vi "电机定位1.1（备份）.vi"(0 "VISA I":refnum<visa-resource-name>, 1 "等待时间(ms)":u32=40, 2 "细分设置":dbl=8.0, 3 "电机急停":bool, 4 "X":dbl, 5 "精度":dbl=0.001, 6 "pulDDR2Length":u32, 8 "hDevice":i32, 10 "M-length":dbl, 12 "N-length":dbl) -> (13 "hDevice out":i32, 14 "VISA O":refnum<visa-resource-name>, 18 "X":dbl, 19 "Y":dbl)   [LabVIEW 2016]
panel:
  out "幅频谱":dbl[](graph)
  out "时域谱":dbl[](graph)
  in  "查询信号":bool
  in  "Y":dbl
  in  "确定":bool
  in  "ESC":bool
  # "时域谱"
  # "频域谱"
  # "目标位置"
  # "实时位置"
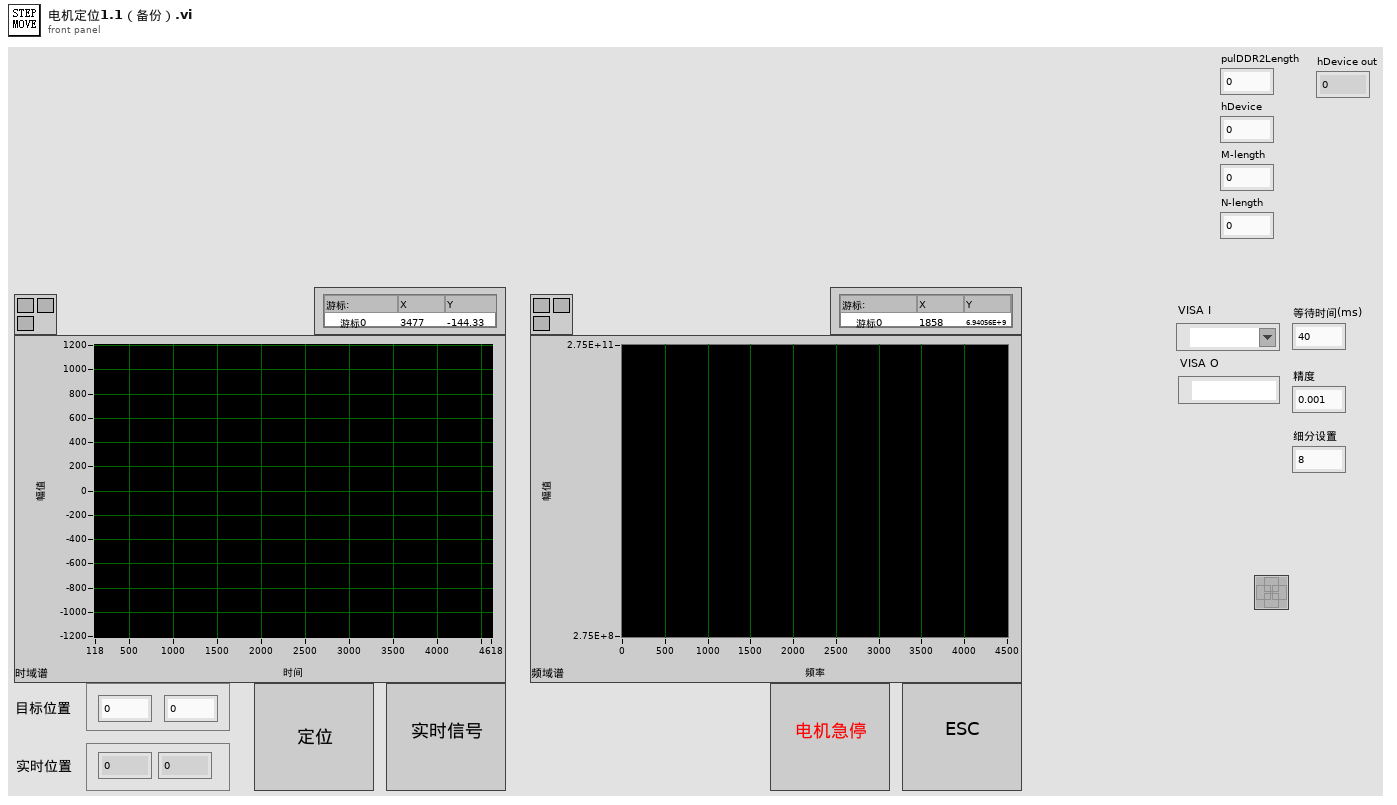
[diagram p1: front panel]
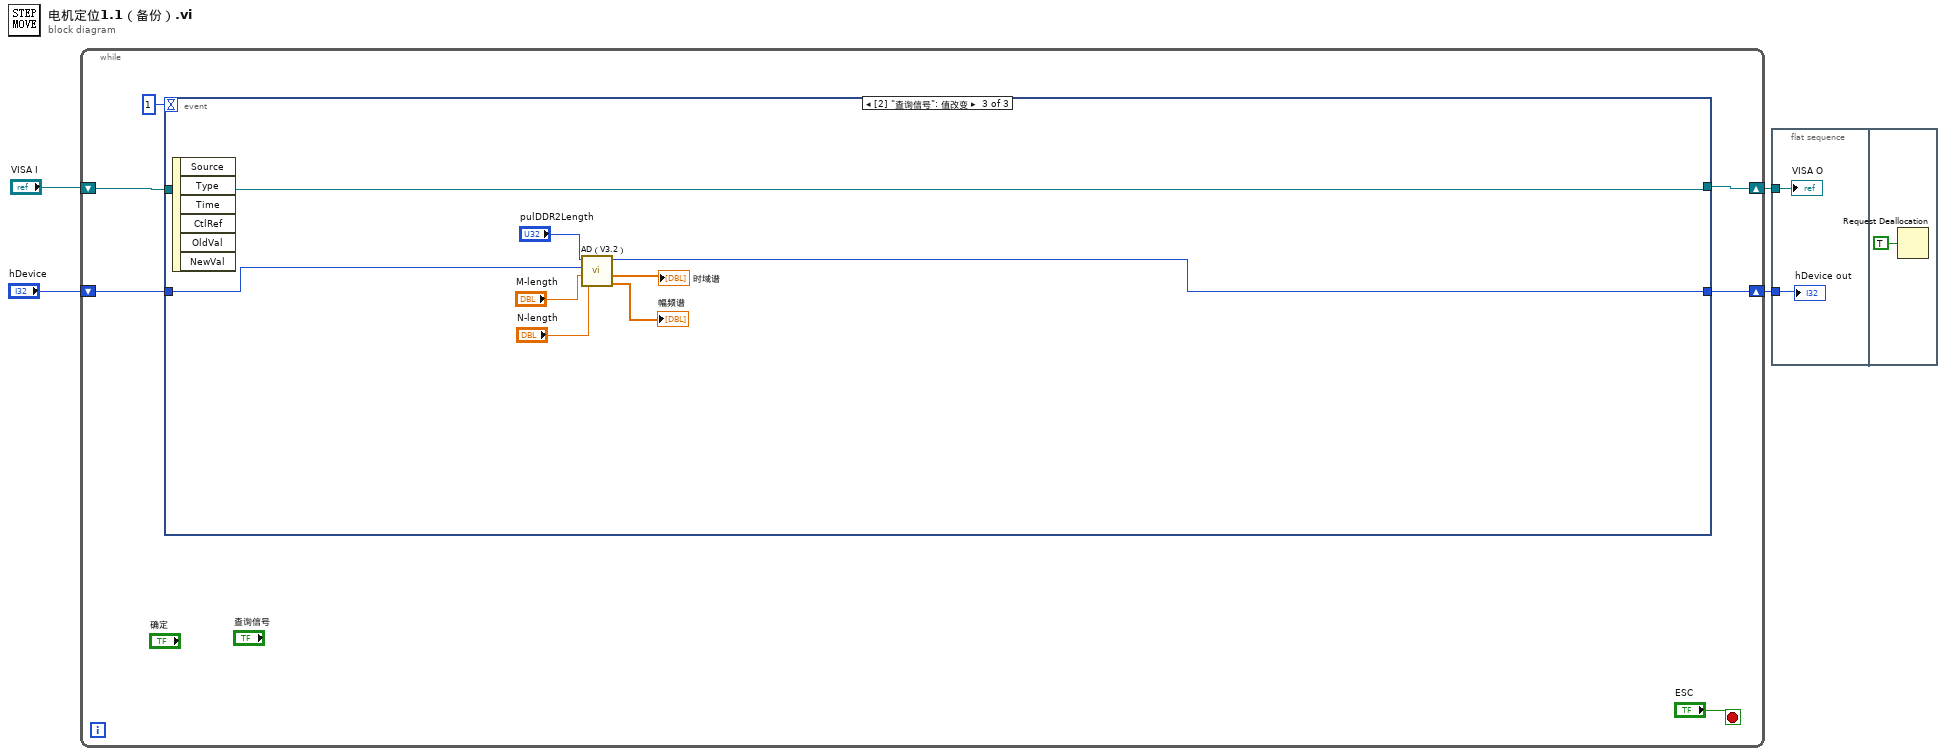
[diagram p0: block diagram]
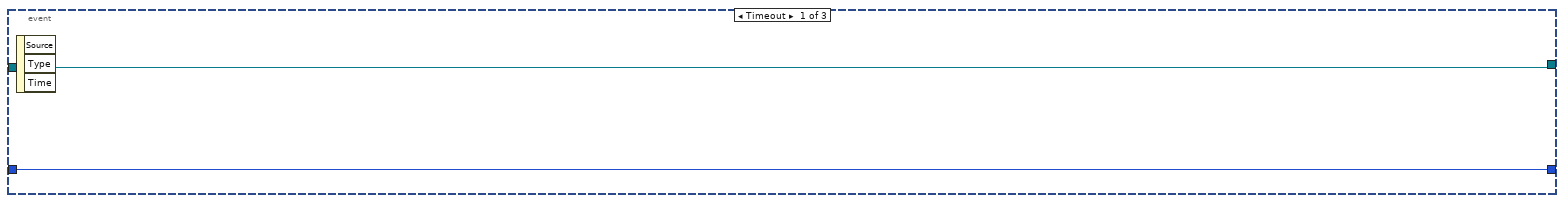
[diagram p2: hidden frame]
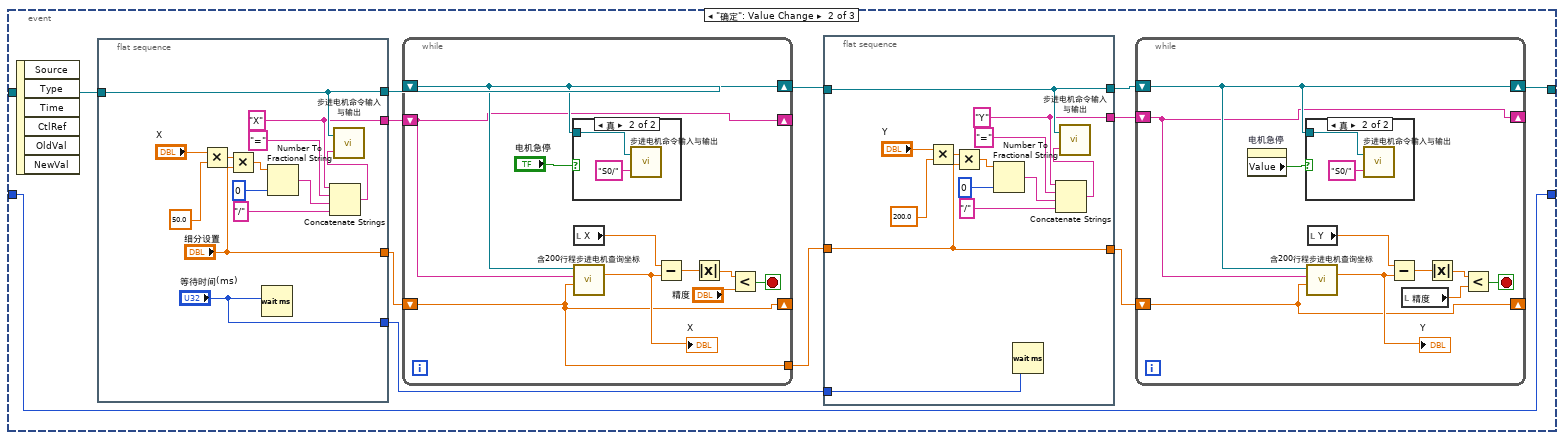
[diagram p3: hidden frame]
diagram:
  n1 = while {
    shift-right: [w9] -> w4
    shift-left: "VISA I" -> [w10]
    shift-right: [w6] -> w1
    shift-left: "hDevice" -> [w7]
    stop <- "ESC" stop-if-true
    n2 = event shown="[2] \"查询信号\": 值改变" {
      selector: _ -> [_ _ _]
      dyn-events: _ -> [_ _ _]
      timeout: 1 -> [_ _ _]
      tunnel: w10 -> [w12 w24 w82]
      tunnel: [w12 w23 w82] -> w9
      tunnel: w7 -> [w11 w13 w76]
      tunnel: [w11 w13 w75] -> w6
      event Timeout {
        n3 = event-data() -> ()  [unwired: 1 in, 3 out]
      }
      event "确定": Value Change {
        n4 = event-data() -> ()  [unwired: 1 in, 6 out]
        n5 = flat-sequence {
          tunnel: w24 -> [w66]
          tunnel: [w66] -> w22
          tunnel: ["细分设置"] -> w21
          tunnel: [w63] -> w20
          tunnel: ["等待时间(ms)"] -> w15
          frame #0 {
            w63 = "X"
            n6 = Multiply(x="X", y=50.0 ("x")) -> (x*y=w69:dbl)
            n7 = Multiply(x=w69, y="细分设置") -> (x*y=w74:dbl)
            n8 = Wait (ms)(milliseconds to wait="等待时间(ms)") -> ()  [unwired: 1 out]
            n9 = Number To Fractional String(number=w74, precision (6)=i16 0 ("精度(6)")) -> (F-format string=w72:string)  [unwired: 2 out]
            n10 = Concatenate Strings(w63, "=" ("字符串"), w72, "/" ("字符串")) -> (w68:string)
            n11 = call "步进电机命令输入与输出.vi"("输入字符串"=w68, "串口通信端口"=w66) -> ()  [unwired: 1 out]
          }
        }
        n12 = while {
          tunnel: [w50] -> w14
          shift-right: [w56] -> w16
          shift-left: w22 -> [w56]
          shift-right: [w51] -> _
          shift-left: w20 -> [w51]
          shift-right: [w50] -> _
          shift-left: w21 -> [w50]
          stop <- w59 stop-if-true
          n13 = case shown="真" "电机急停" {
            tunnel: w56 -> [_ w60]
            frame False {
            }
            frame True {
              n14 = call "步进电机命令输入与输出.vi"("输入字符串"="S0/", "串口通信端口"=w60) -> ()  [unwired: 1 out]
            }
          }
          n15 = local read "X"() -> (w54:dbl)
          n16 = call "含200行程步进电机查询坐标.vi"("细分设置"=w50, "查询坐标轴"=w51, "串口通信端口"=w56) -> ("坐标(mm)"=w53:dbl)  [unwired: 8 in]
          "X" <- w53
          n17 = Subtract(x=w54, y=w53) -> (x-y=w58:dbl)
          n18 = Absolute Value(x=w58) -> (abs(x)=w57:dbl)
          n19 = Less?(x=w57, y="精度") -> (x < y?=w59:bool)
        }
        n20 = flat-sequence {
          tunnel: w16 -> [w41]
          tunnel: [w41] -> w19
          tunnel: [w37] -> w18
          tunnel: [w39] -> w17
          tunnel: w15 -> [w38]
          tunnel: w14 -> [w37]
          frame #0 {
            w39 = "Y"
            n21 = Multiply(x="Y", y=200.0 ("x")) -> (x*y=w44:dbl)
            n22 = Multiply(x=w44, y=w37) -> (x*y=w49:dbl)
            n23 = Number To Fractional String(number=w49, precision (6)=i16 0 ("精度(6)")) -> (F-format string=w47:string)  [unwired: 2 out]
            n24 = Wait (ms)(milliseconds to wait=w38) -> ()  [unwired: 1 out]
            n25 = Concatenate Strings(w39, "=" ("字符串"), w47, "/" ("字符串")) -> (w43:string)
            n26 = call "步进电机命令输入与输出.vi"("输入字符串"=w43, "串口通信端口"=w41) -> ()  [unwired: 1 out]
          }
        }
        n27 = while {
          shift-right: [w31] -> w23
          shift-left: w19 -> [w31]
          shift-right: [w26] -> _
          shift-left: w17 -> [w26]
          shift-right: [w25] -> _
          shift-left: w18 -> [w25]
          stop <- w34 stop-if-true
          n28 = property on="电机急停" class="Bool (严格)"() -> ("Value"=w27:bool)  [unwired: 2 in, 2 out]
          n29 = case shown="真" w27 {
            tunnel: w31 -> [_ w35]
            frame False {
            }
            frame True {
              n30 = call "步进电机命令输入与输出.vi"("输入字符串"="S0/", "串口通信端口"=w35) -> ()  [unwired: 1 out]
            }
          }
          n31 = call "含200行程步进电机查询坐标.vi"("细分设置"=w25, "查询坐标轴"=w26, "串口通信端口"=w31) -> ("坐标(mm)"=w29:dbl)  [unwired: 8 in]
          "Y" <- w29
          n32 = local read "Y"() -> (w30:dbl)
          n33 = Subtract(x=w30, y=w29) -> (x-y=w33:dbl)
          n34 = local read "精度"() -> (w28:dbl)
          n35 = Absolute Value(x=w33) -> (abs(x)=w32:dbl)
          n36 = Less?(x=w32, y=w28) -> (x < y?=w34:bool)
        }
      }
      event "查询信号": Value Change {
        n37 = event-data() -> ()  [unwired: 1 in, 6 out]
        n38 = call "AD（V3.2）.vi"("N-length"="N-length", "M-length"="M-length", "hDevice"=w76, "pulDDR2Length"="pulDDR2Length") -> ("幅频谱"=→"幅频谱":dbl[], "时域谱"=→"时域谱":dbl[], "hDevice out"=w75:i32)  [unwired: 5 in]
      }
    }
  }
  n39 = flat-sequence {
    tunnel: w4 -> [w84]
    tunnel: w1 -> [w83]
    frame #0 {
      "VISA O" <- w84
      "hDevice out" <- w83
    }
    frame #1 {
      n40 = Request Deallocation(TRUE ("标志")) -> ()
    }
  }
